vi "Acc G test2.vi"() -> ()   [LabVIEW 2013]
panel:
  out "Y max":dbl caption="Y 최대" format="%0.2f"
  in  "웨이브폼 그래프":waveform(dbl)[](graph)
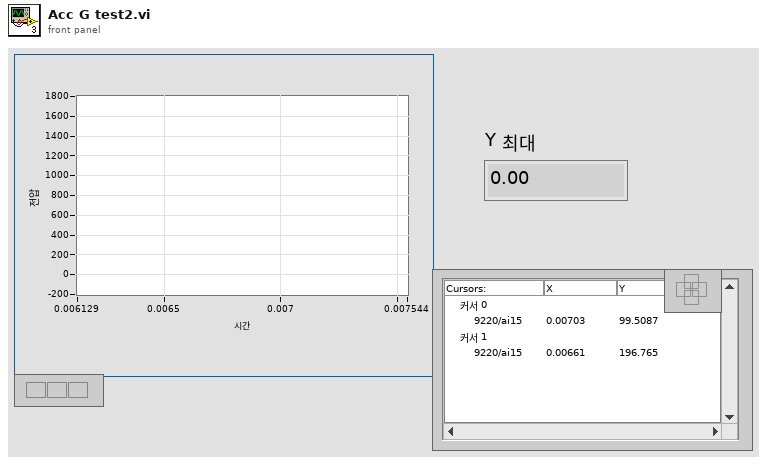
[diagram p1: front panel]
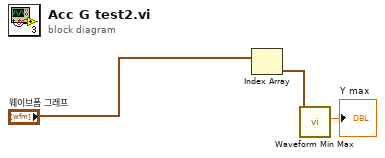
[diagram p0: block diagram]
diagram:
  n1 = Index Array(array="웨이브폼 그래프") -> (element=w3:waveform(dbl))  [unwired: 1 in]
  n2 = call <vilib>:"Waveform Min Max.vi"("waveform in"=w3) -> ("Y max"=→"Y max":dbl)  [unwired: 5 in, 5 out]
